vi "Set Value Write.vi"(8 "error in (no error)":errorcluster caption="entrée d'erreur (pas d'erreur)", 10 "Value Write":bool, 11 "Class DIO en entrée":refnum<class "Class Instrument DIO.lvclass">) -> (0 "error out":errorcluster caption="sortie d'erreur", 3 "Class DIO en Sortie":refnum<class "Class Instrument DIO.lvclass">)   [LabVIEW 2020, in "Library Instrument & Equipement.lvlib" / "Library Instruments.lvlib" / "Class Instrument DIO.lvclass"]
uses:
  Class Instrument DIO.lvclass
  Class Instrument DIO.lvclass/Class Instrument DIO.ctl
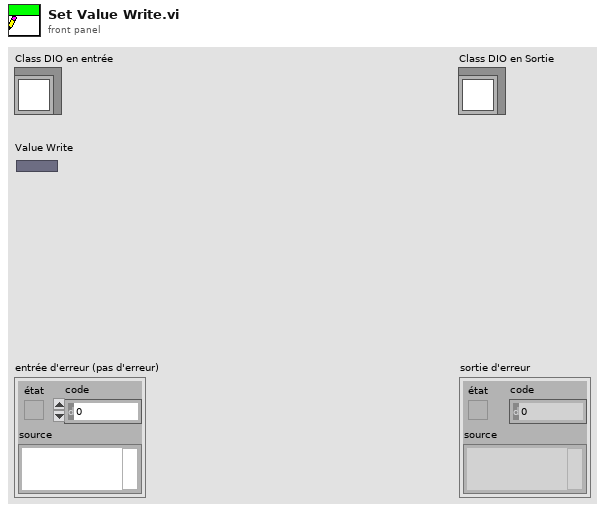
[diagram p1: front panel]
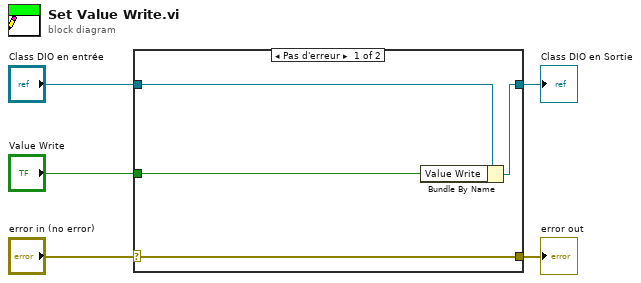
[diagram p0: block diagram]
diagram:
  n1 = case shown="Pas d'erreur" "error in (no error)" {
    selector: "error in (no error)" -> [w9 w10]
    tunnel: [w9 w10] -> w4
    tunnel: [w7 w11] -> w2
    tunnel: "Class DIO en entrée" -> [w8 w11]
    tunnel: "Value Write" -> [w6 _]
    frame No Error {
      n2 = Bundle By Name(cluster=w8, "Value Write"=w6) -> (w7:refnum<class "Class Instrument DIO.lvclass">)
    }
    frame Error {
    }
  }
  "error out" <- w4
  "Class DIO en Sortie" <- w2
